vi "_Fade(String).vi"(6 "Fade (Exponential)":T1, 8 "error in":errorcluster, 9 "Target Transparency (0)":u8, 10 "Fade time (ms)":string, 11 "VI Reference (calling VI)":refnum<vi>) -> (0 "error out":errorcluster, 3 "dup VI Reference":refnum<vi>)   [LabVIEW 2012]
doc: "Produces a fade in or out, from the actual value to the target transparency. Use this generic VI when you start from an unknown transparency value.\n\nString input is provided to be used with string-based state machines."
uses:
  _fadetype.ctl
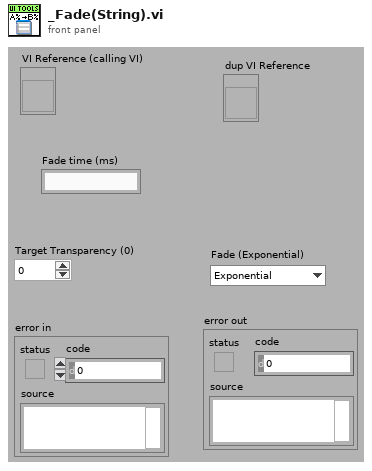
[diagram p1: front panel]
types:
  T1 = typedef "_fadetype.ctl" = enum16{"Exponential", "Linear"}
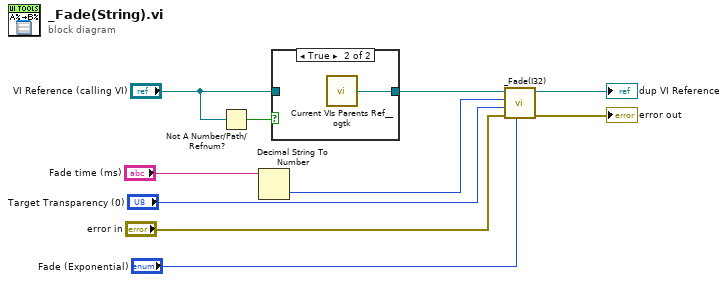
[diagram p0: block diagram]
diagram:
  n1 = Not A Number/Path/Refnum?(number/path/refnum="VI Reference (calling VI)") -> (NaN/Path/Refnum?=w10:bool)
  n2 = Decimal String To Number(string="Fade time (ms)") -> (number=w1:i32)  [unwired: 3 out]
  n3 = case shown="True" w10 {
    tunnel: "VI Reference (calling VI)" -> [w11 _]
    tunnel: [w11 w12] -> w6
    frame False {
    }
    frame True {
      n4 = call <userlib>:"Current VIs Parents Ref__ogtk.vi"() -> ("Calling VI's Reference"=w12:refnum<vi>)  [unwired: 2 out]
    }
  }
  n5 = call "_Fade(I32).vi"("Fade (Exponential)"="Fade (Exponential)", "error in"="error in", "Target Transparency (0)"="Target Transparency (0)", "Fade time (ms)"=w1, "VI Reference (calling VI)"=w6) -> ("error out"=→"error out":errorcluster, "dup VI Reference"=→"dup VI Reference":refnum<vi>)  [unwired: 5 out]
